vi "Get LDF Frame and Sched(IL).vi"(8 "error in (no error)":errorcluster, 11 "LDF Path":path) -> (0 "error out":errorcluster, 3 "LIN Device":T1={"Master Frame(3C)"="MasterReq\nSPA3414_ConfigurationsCMAGeely_CEMCALYPSOSDB34XX0Cfg_LIN3_190709_", "Slave Frame(3D)"="SlaveResp\nSPA3414_ConfigurationsCMAGeely_CEMCALYPSOSDB34XX0Cfg_LIN3_190709_", "Request Schedule"="CEMLIN3DiagRequestSchedule\nSPA3414_ConfigurationsCMAGeely_CEMCALYPSOSDB34XX0Cfg_LIN3_190709_", "Response Schedule"="CEMLIN3DiagResponseSchedule\nSPA3414_ConfigurationsCMAGeely_CEMCALYPSOSDB34XX0Cfg_LIN3_190709_", "Frame Write SCU"="", "Frame Read SCU"="", "LIN Name"=""})   [LabVIEW 2018]
uses:
  LIN Device.ctl
  <resource>/objmgr/xnet.rc
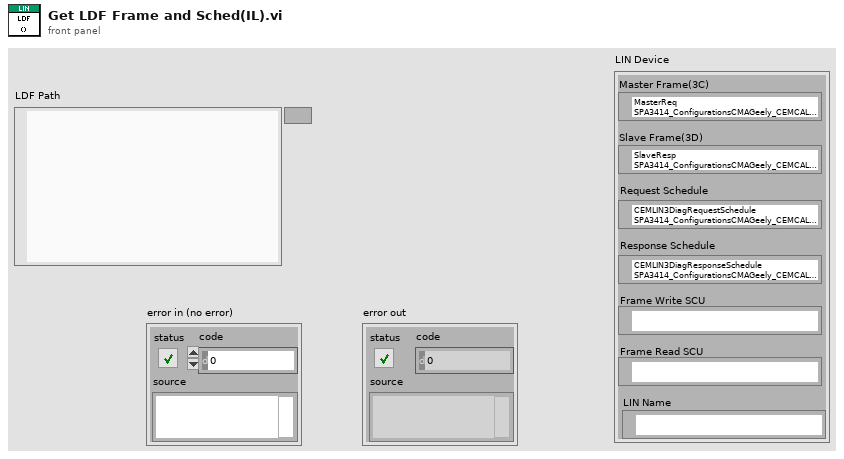
[diagram p1: front panel]
types:
  T1 = typedef "LIN Device.ctl" = cluster{"Master Frame(3C)":refnum<k21>, "Slave Frame(3D)":refnum<k21>, "Request Schedule":refnum<k21>, "Response Schedule":refnum<k21>, "Frame Write SCU":refnum<k21>, "Frame Read SCU":refnum<k21>, "LIN Name":refnum<k21>}
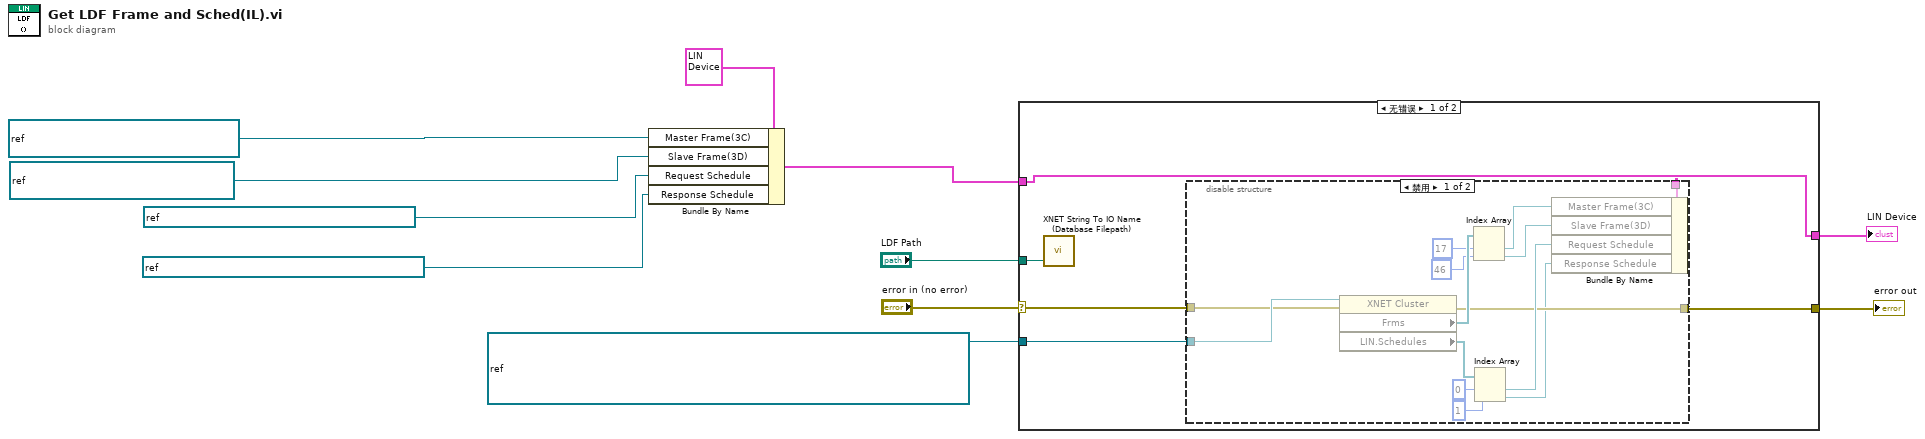
[diagram p0: block diagram]
diagram:
  n1 = Bundle By Name(cluster=T1 {"Master Frame(3C)"="MasterReq\nSPA3414_ConfigurationsCMAGeely_CEMCALYPSOSDB34XX0Cfg_LIN3_190709_", "Slave Frame(3D)"="SlaveResp\nSPA3414_ConfigurationsCMAGeely_CEMCALYPSOSDB34XX0Cfg_LIN3_190709_", "Request Schedule"="CEMLIN3DiagRequestSchedule\nSPA3414_ConfigurationsCMAGeely_CEMCALYPSOSDB34XX0Cfg_LIN3_190709_", "Response Schedule"="CEMLIN3DiagResponseSchedule\nSPA3414_ConfigurationsCMAGeely_CEMCALYPSOSDB34XX0Cfg_LIN3_190709_", "Frame Write SCU"="", "Frame Read SCU"="", "LIN Name"=""} ("LIN Device"), "Master Frame(3C)"=refnum<k21> "MasterReq\nCD701_CEM_LIN3_20230222", "Slave Frame(3D)"=refnum<k21> "SlaveResp\nCD701_CEM_LIN3_20230222" ("Master Frame(3C)"), "Request Schedule"=refnum<k21> "Cem_Lin3DiagRequestSchedule_CEM_LIN3\nCD701_CEM_LIN3_20230222", "Response Schedule"=refnum<k21> "Cem_Lin3DiagResponseSchedule_CEM_LIN3\nCD701_CEM_LIN3_20230222" ("Request Schedule")) -> (w7:T1)
  n2 = case shown="无错误" "error in (no error)" {
    selector: "error in (no error)" -> [w13 w33]
    tunnel: "LDF Path" -> [w16 _]
    tunnel: [w15 w33] -> w9
    tunnel: refnum<k21> "SPA3414_ConfigurationsCMAGeely_CEMCALYPSOSDB34XX0Cfg_LIN3_190709_" ("element") -> [w14 _]
    tunnel: [w12 w32] -> w1
    tunnel: w7 -> [w12 w32]
    frame No Error {
      n3 = call <vilib>:"XNET String To IO Name (Database Filepath).vi"("filepath"=w16) -> ()  [unwired: 4 in, 1 out]
      n4 = disable-structure shown="禁用" {
        disable-tunnel: [w21 w31] -> w15
        disable-tunnel: w14 -> [w19 _]
        disable-tunnel: w13 -> [w18 w31]
        disable-tunnel: _ -> [w17 _]
        frame Disabled {
          n5 = property class="XNET Cluster"(reference=w19, error in=w18) -> (error out=w21:errorcluster, "Frms"=w30:refnum<k21>[], "LIN.Schedules"=w27:refnum<k21>[])  [unwired: 1 out]
          n6 = Index Array(array=w30, index #1=17 ("index"), index #2=46 ("index")) -> (element #1=w24:refnum<k21>, element #2=w23:refnum<k21>)
          n7 = Index Array(array=w27, index #1=0 ("index"), index #2=1 ("index")) -> (element #1=w22:refnum<k21>, element #2=w20:refnum<k21>)
          n8 = Bundle By Name(cluster=w17, "Master Frame(3C)"=w24, "Slave Frame(3D)"=w23, "Request Schedule"=w22, "Response Schedule"=w20) -> ()  [unwired: 1 out]
        }
        frame Enabled {
        }
      }
    }
    frame Error {
    }
  }
  "error out" <- w9
  "LIN Device" <- w1
